vi "svfa_Average Array (complex) No State.vi"(6 "averaging state info in":T2={"complex FFT"=[], "real FFT"=[], "f0"=0.0, "df"=0.0, "averages completed"=0.0, "averaging parameters"={"averaging mode"=enum."No averaging", "weighting mode"=enum."Linear", "number of averages"=10, "linear mode"=enum."Auto restart"}} {"averages completed" format="%.2f"; "df" format="%.2f"; "f0" format="%.2f"; "real FFT" format="%.2f"; "complex FFT" format="%.2f"}, 7 "processing control":T1(ring), 11 "array":cdb[](array[numeric]) format="%.2f") -> (0 "averages completed":dbl, 1 "averaging done":bool, 3 "average array":cdb[](array[numeric]) format="%.2f", 4 "averaging state info out":T3={"complex FFT"=[], "Mag/Real FFT"=[], "f0"=0.0, "df"=0.0, "averages completed"=0.0, "averaging parameters"={"averaging mode"=enum."No averaging", "weighting mode"=enum."Linear", "number of averages"=10, "linear mode"=enum."Auto restart"}} {"averages completed" format="%.2f"; "df" format="%.2f"; "f0" format="%.2f"; "Mag/Real FFT" format="%.2f"; "complex FFT" format="%.2f"})   [LabVIEW 2017]
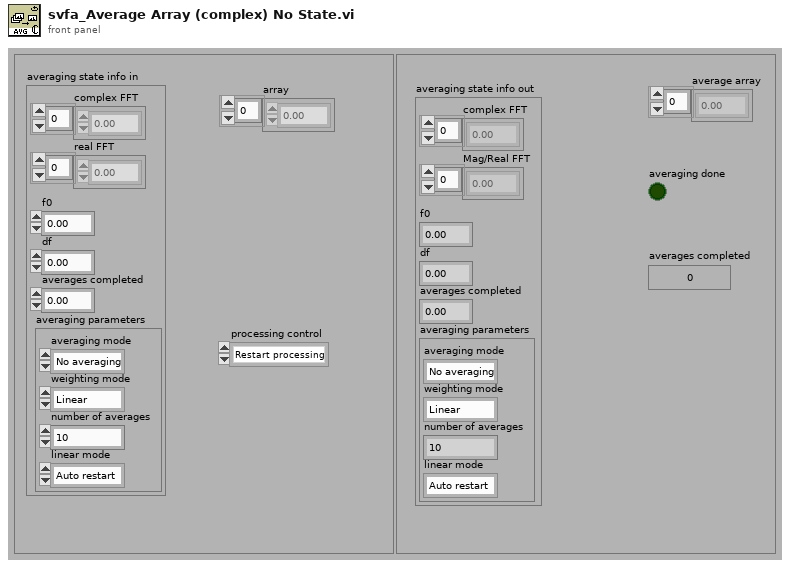
[diagram p1: front panel]
types:
  T1 = enum16{"Restart processing", "Continue processing", "Skip processing"}
  T2 = cluster{"complex FFT":cdb[], "real FFT":dbl[], "f0":dbl, "df":dbl, "averages completed":dbl, "averaging parameters":cluster{"averaging mode":enum16{"No averaging", "Vector averaging", "RMS averaging", "Peak hold"}, "weighting mode":enum16{"Linear", "Exponential"}, "number of averages":u32, "linear mode":enum16{"One shot", "Auto restart"}}}
  T3 = cluster{"complex FFT":cdb[], "Mag/Real FFT":dbl[], "f0":dbl, "df":dbl, "averages completed":dbl, "averaging parameters":cluster{"averaging mode":enum16{"No averaging", "Vector averaging", "RMS averaging", "Peak hold"}, "weighting mode":enum16{"Linear", "Exponential"}, "number of averages":u32, "linear mode":enum16{"One shot", "Auto restart"}}}
  T4 = enum16{"No averaging", "Vector averaging", "RMS averaging", "Peak hold"}
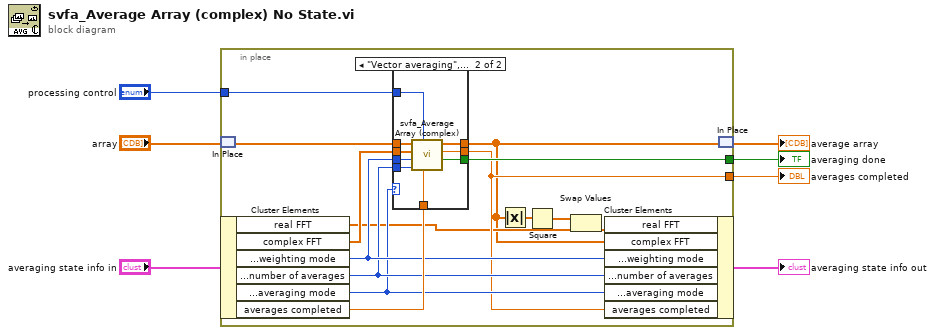
[diagram p0: block diagram]
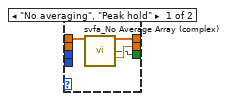
[diagram p2: hidden frame]
diagram:
  n1 = in-place {
    in-place-border: [w14] -> w7
    in-place-border: [w21] -> w6
    in-place-border: "processing control" -> [w20]
    n2 = in-place-match #1("array") -> (w13:cdb[])
    n3 = in-place-cluster #2("averaging state info in") -> ("real FFT"=w12:dbl[], "complex FFT"=w19:cdb[], "averaging parameters.weighting mode"=w17:enum16{"Linear", "Exponential"}, "averaging parameters.number of averages"=w16:u32, "averaging parameters.averaging mode"=w15:T4, "averages completed"=w18:dbl)
    n4 = case shown="\"Vector averaging\", \"RMS averaging\", Default" w15 {
      tunnel: [w23 w34] -> w14
      tunnel: w19 -> [_ w33]
      tunnel: w13 -> [w25 w32]
      tunnel: [w22 w31] -> w21
      tunnel: w18 -> [_ w30]
      tunnel: w17 -> [_ w29]
      tunnel: w16 -> [_ w28]
      tunnel: w20 -> [_ w27]
      tunnel: [w24 w26] -> w9
      frame "No averaging", "Peak hold" {
        n5 = call <vilib>:"svfa_No Average Array (complex).vi"("array"=w25) -> ("dup array"=w24:cdb[], "averaging done"=w22:bool, "averages completed"=w23:dbl)  [unwired: 10 in, 2 out]
      }
      frame "Vector averaging", "RMS averaging", Default {
        n6 = call <vilib>:"svfa_Average Array (complex).vi"("averages completed in"=w30, "processing control"=w27, "number of averages"=w28, "weighting mode"=w29, "previous average array"=w33, "array"=w32) -> ("averaging done"=w31:bool, "averages completed out"=w34:dbl, "average array"=w26:cdb[])  [unwired: 3 in]
      }
    }
    n7 = Absolute Value(x=w9) -> (abs(x)=w11:dbl[])
    n8 = Square(x=w11) -> (x^2=w8:dbl[])
    n9 = Swap Values(12:w8, 14:w12) -> (3:w10:dbl[])  [unwired: 1 in, 1 out]
    n10 = in-place-cluster #2("real FFT"=w10, "complex FFT"=w9, "averaging parameters.weighting mode"=w17, "averaging parameters.number of averages"=w16, "averaging parameters.averaging mode"=w15, "averages completed"=w14) -> (→"averaging state info out":T2)
    n11 = in-place-match #1(w9) -> (→"average array":cdb[])
  }
  "averages completed" <- w7
  "averaging done" <- w6
